vi "Power Off.vi"(8 "error in (no error)":errorcluster, 11 "Dual Fan in":refnum<class "Dual Fan.lvclass">) -> (0 "error out":errorcluster, 3 "Dual Fan out":refnum<class "Dual Fan.lvclass">)   [LabVIEW 2015, in "Dual Fan.lvlib" / "Dual Fan.lvclass"]
uses:
  Dual Fan.lvclass
  Dual Fan.lvclass/Dual Fan.ctl
  Simulation/Simulation Data_Global.vi
  Simulation/Simulation.lvlib
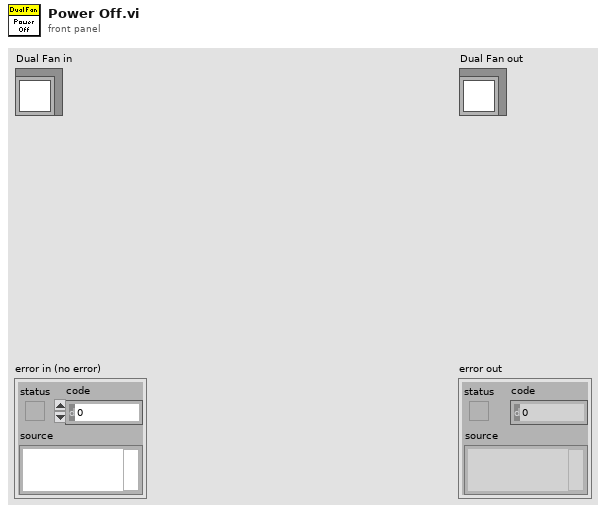
[diagram p1: front panel]
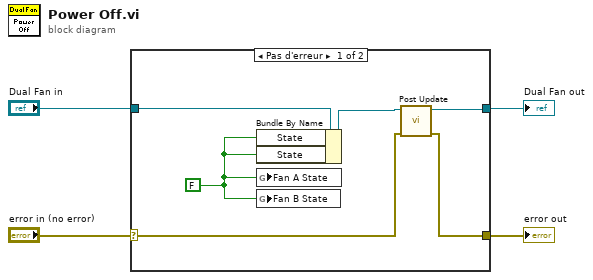
[diagram p0: block diagram]
diagram:
  n1 = case shown="Pas d'erreur" "error in (no error)" {
    selector: "error in (no error)" -> [w6 w12]
    tunnel: [w5 w12] -> w3
    tunnel: [w7 w11] -> w1
    tunnel: "Dual Fan in" -> [w10 w11]
    frame No Error {
      w9 = FALSE ("Fan A State")
      n2 = Bundle By Name(cluster=w10, "State"=w9, "State"=w9) -> (w8:refnum<class "Dual Fan.lvclass">)
      n3 = global write "Simulation Data_Global.vi" "Fan A State"(w9) -> ()
      n4 = global write "Simulation Data_Global.vi" "Fan B State"(w9) -> ()
      n5 = call "Post Update.vi"("error in (no error)"=w6, "Dual Fan in"=w8) -> ("error out"=w5:errorcluster, "Dual Fan out"=w7:refnum<class "Dual Fan.lvclass">)  [unwired: 8 in]
    }
    frame Error {
    }
  }
  "error out" <- w3
  "Dual Fan out" <- w1
